vi "Begin.vi"() -> (1 "CameraDevRef":T1)   [LabVIEW 2011]
doc: "Called before other user functions, this VI is expected to open initial I/O refnums, load in file data, and do all program initialization. Notice that the <B>error out</B> terminal is simply used for data flow. Wiring it to other structures or subVIs ensures that this VI runs first."
uses:
  <vilib>/Rock Robotics/WPI/Camera/WPI_CameraDevRef.ctl
  <vilib>/Rock Robotics/SystemInterfaces/DIO/FPGA_DIOPWMChannel.ctl
  <vilib>/Rock Robotics/WPI/Joystick/WPI_JoystickDeviceEnum.ctl
  <vilib>/Rock Robotics/SystemInterfaces/AI/FPGA_AIChannel.ctl
  <vilib>/Rock Robotics/SystemInterfaces/DIO/FPGA_DIORelayChannel.ctl
  <vilib>/Rock Robotics/SystemInterfaces/DIO/FPGA_DIOChannel.ctl
  <vilib>/Rock Robotics/SystemInterfaces/AI/FPGA_AIGyroChannel.ctl
  <vilib>/Rock Robotics/WPI/Encoder/WPI_EncoderType.ctl
  <vilib>/Rock Robotics/WPI/MotorControl/WPI_MotorControlOpen Jaguar.vi
  Robot Global Data.vi
  <vilib>/Utility/file.llb/Read From Spreadsheet File (DBL).vi
  <vilib>/Rock Robotics/WPI/Counter/WPI_CounterDigitalInputToDigitalSource.vi
  <vilib>/Rock Robotics/WPI/RobotDrive/WPI_RobotDriveOpen2MotorWithVictor.vi
  <vilib>/Rock Robotics/WPI/Relay/WPI_RelayDirection.ctl
  <vilib>/Rock Robotics/SystemInterfaces/Typedef/FPGA_TypedefDigitalModule.ctl
  <vilib>/Rock Robotics/SystemInterfaces/Typedef/FPGA_TypedefAnalogModule.ctl
  <vilib>/Rock Robotics/WPI/MotorControl/WPI_MotorControlOpen Victor.vi
panel:
  in  "Minimum Rate":dbl=20.0
  in  "Number Samples to Average":u8=1 min=1 max=128
  in  "DistancePerCount":dbl=1.0
  out "data from file":dbl[](graph)
  in  "Scripted":bool
  out "Path and file":string
  in  "Balls In Robot At Start":dbl
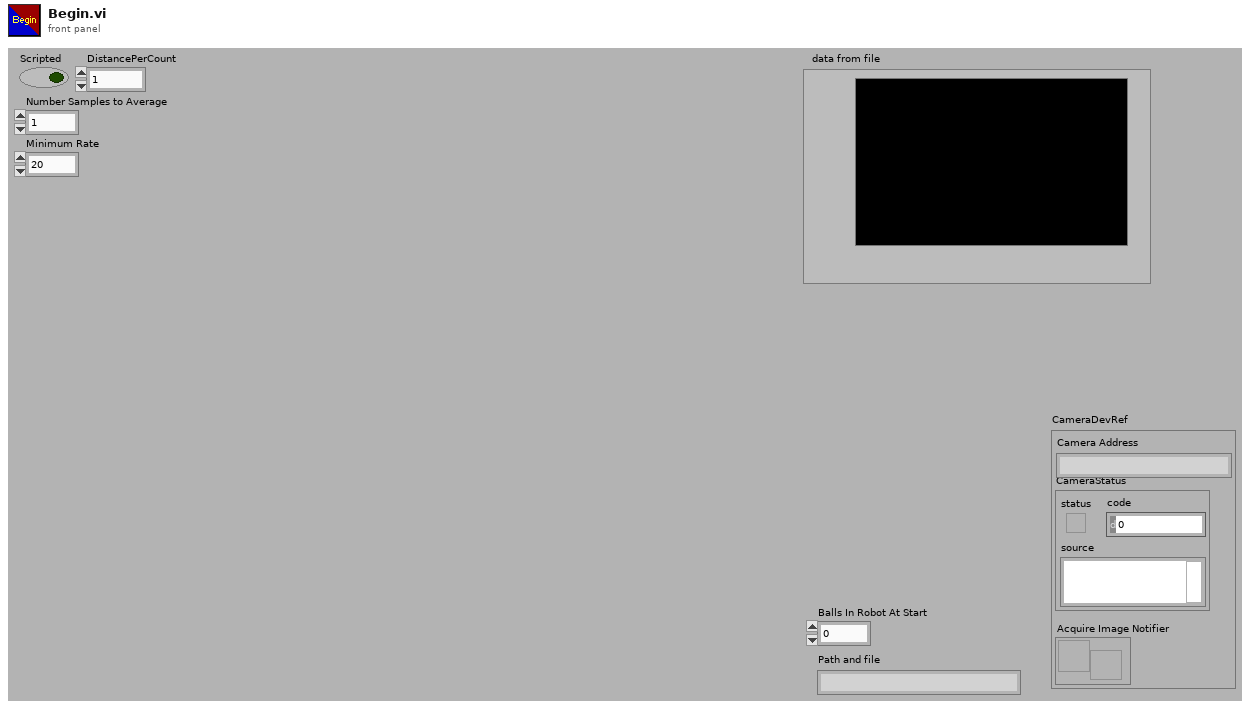
[diagram p1: front panel]
types:
  T1 = typedef "WPI_CameraDevRef.ctl" = cluster{"Camera Address":string, "CameraStatus":errorcluster, "Acquire Image Notifier":refnum<notifier>}
  T2 = typedef "WPI_EncoderType.ctl" = enum16{"1x", "2x", "4x"}
  T3 = typedef "FPGA_DIOChannel.ctl" = enum8{"DIO 1", "DIO 2", "DIO 3", "DIO 4", "DIO 5", "DIO 6", "DIO 7", "DIO 8", "DIO 9", "DIO 10", "DIO 11", "DIO 12", "DIO 13", "DIO 14", "Invalid"}
  T4 = typedef "FPGA_AIGyroChannel.ctl" = enum8{"AI 1", "AI 2", "Invalid"}
  T5 = typedef "FPGA_DIOPWMChannel.ctl" = enum8{"PWM 1", "PWM 2", "PWM 3", "PWM 4", "PWM 5", "PWM 6", "PWM 7", "PWM 8", "PWM 9", "PWM 10", "Invalid"}
  T6 = typedef "FPGA_DIORelayChannel.ctl" = enum8{"Relay 1", "Relay 2", "Relay 3", "Relay 4", "Relay 5", "Relay 6", "Relay 7", "Relay 8", "Invalid"}
  T7 = typedef "FPGA_AIChannel.ctl" = enum8{"AI 1", "AI 2", "AI 3", "AI 4", "AI 5", "AI 6", "AI 7", "AI 8", "Invalid"}
  T8 = typedef "WPI_JoystickDeviceEnum.ctl" = enum16{"USB 1", "USB 2", "USB 3", "USB 4", "Kinect 1", "Kinect 2"}
  T9 = typedef "WPI_MotorControlDeviceRef.ctl" = cluster{"DeviceStatus":errorcluster, "Type":enum16{"PWM", "CAN"}, "PWM":cluster{"Digital Module":T10, "PWM Channel":T5, "DeadBand":T11}, "CAN":cluster{"Device Number":u8, "Control Mode":T12, "Semaphore":T13, "Max Vout":dbl}, "Invert":bool, "TransformRef":T14, "InvTransformRef":T14}
  T10 = typedef "FPGA_TypedefDigitalModule.ctl" = enum16{"Digital Module 1", "Digital Module 2"}
  T11 = typedef "WPI_PWMDeadband.ctl" = cluster{"Name":string, "maxPositivePwm":i32, "minPositivePwm":i32, "centerPwm":i32, "maxNegativePwm":i32, "minNegativePwm":i32, "angularRange":u16}
  T12 = typedef "WPI_CANJaguar_ControlMode.ctl" = enum8{"Percent VBus", "Current", "Speed", "Position", "Voltage"}
  T13 = typedef "Semaphore RefNum" = refnum<k1>
  T14 = typedef "WPI_PWMTransform_ConPane.ctl" = refnum<vi>
  T15 = typedef "WPI_RobotDriveDevRef.ctl" = cluster{"DevStatus":errorcluster, "Motors[]":T9[], "Square Inputs":bool, "Max Output":dbl, "Isochronous":bool}
  T16 = typedef "WPI_CameraImageSize.ctl" = enum16{"640x480", "320x240", "160x120"}
  T17 = cluster{"fps":i32, "compression":i32, "Image Size":T16}
  T18 = typedef "WPI_AnalogChannelDevRef.ctl" = cluster{"DevStatus":errorcluster, "Analog Module":T19, "Analog Channel":T7}
  T19 = typedef "FPGA_TypedefAnalogModule.ctl" = enum16{"Analog Module 1", "Analog Module 2"}
  T20 = typedef "WPI_ServoDeviceRef.ctl" = cluster{"DeviceStatus":errorcluster, "Digital Module":T10, "PWM Channel":T5, "DeadBand":T11}
  T21 = typedef "WPI_CameraWhite Balance Values.ctl" = enum16{"Auto", "Fixed indoor", "Fixed outdoor 1", "Fixed outdoor 2", "Fixed fluorescent 1", "Fixed fluorescent 2", "Hold current"}
  T22 = typedef "WPI_RelayDirection.ctl" = enum16{"Both directions", "Forward only", "Reverse only"}
  T23 = typedef "WPI_RelayDevRef.ctl" = cluster{"DevStatus":errorcluster, "Relay Channel":T6, "Digital Module":T10, "Relay Direction":T22}
  T24 = typedef "WPI_JoystickDevRef.ctl" = cluster{"Device":T8}
  T25 = typedef "WPI_CameraExposure Values.ctl" = enum16{"Auto", "Flicker-free 50 Hz", "Flicker-free 60 Hz", "Hold current"}
  T26 = typedef "WPI_DigitalInputDevRef.ctl" = cluster{"DevStatus":errorcluster, "DIO Channel":T3, "Digital Module":T10}
  T27 = typedef "FPGA_CounterEncoderSourceConvertionLVSourceType.ctl" = cluster{"DevStatus":errorcluster, "AnalogTriggerMode?":bool, "DigitalMode":cluster{"Digital Module":T10, "DIO Channel":T28}, "AnalogTriggerMode":cluster{"AnalogTriggerIndex":T29, "OutputType":T30}}
  T28 = typedef "FPGA_DIODigitalSourceChannel.ctl" = enum8{"DIO 1", "DIO 2", "DIO 3", "DIO 4", "DIO 5", "DIO 6", "DIO 7", "DIO 8", "DIO 9", "DIO 10", "DIO 11", "DIO 12", "DIO 13", "DIO 14", "Disabled"}
  T29 = typedef "FPGA_AnalogTriggerIndex.ctl" = enum8{"Trig 0", "Trig 1", "Trig 2", "Trig 3", "Trig 4", "Trig 5", "Trig 6", "Trig 7", "Invalid"}
  T30 = typedef "FPGA_AnalogTriggerOutType.ctl" = enum16{"InWindow", "TriggerState", "Rising", "Falling"}
  T31 = typedef "WPI_EncoderDevRef.ctl" = cluster{"DevStatus":errorcluster, "EncoderIndex":T32, "CounterIndex":T33, "DistancePerCount":dbl, "Decoding Type":T2}
  T32 = typedef "FPGA_EncoderIdx.ctl" = enum8{"Enc 0", "Enc 1", "Enc 2", "Enc 3", "Invalid"}
  T33 = typedef "FPGA_CounterCtrSystemIndex.ctl" = enum8{"Ctr 0", "Ctr 1", "Ctr 2", "Ctr 3", "Ctr 4", "Ctr 5", "Ctr 6", "Ctr 7", "Invalid"}
  T34 = enum16{"big-endian, network order", "native, host order", "little-endian"}
  T35 = cluster{"[0]":dbl, "[1]":dbl, "[2]":dbl, "[3]":dbl, "[4]":dbl, "[5]":dbl, "[6]":dbl, "[7]":dbl, "[8]":dbl}
  T36 = typedef "WPI_GyroDevRef.ctl" = cluster{"DevStatus":errorcluster, "Analog Module":T19, "Analog Channel":T7, "Offset":dbl, "Gain (VoltsPerDegree/Second)":dbl}
  T37 = typedef "WPI_UltrasonicDeviceRef.ctl" = cluster{"DevStatus":errorcluster, "Ping Digital Module":T10, "Echo Digital Module":T10, "Ping Channel":T3, "Echo Channel":T3, "CntIndex":T33}
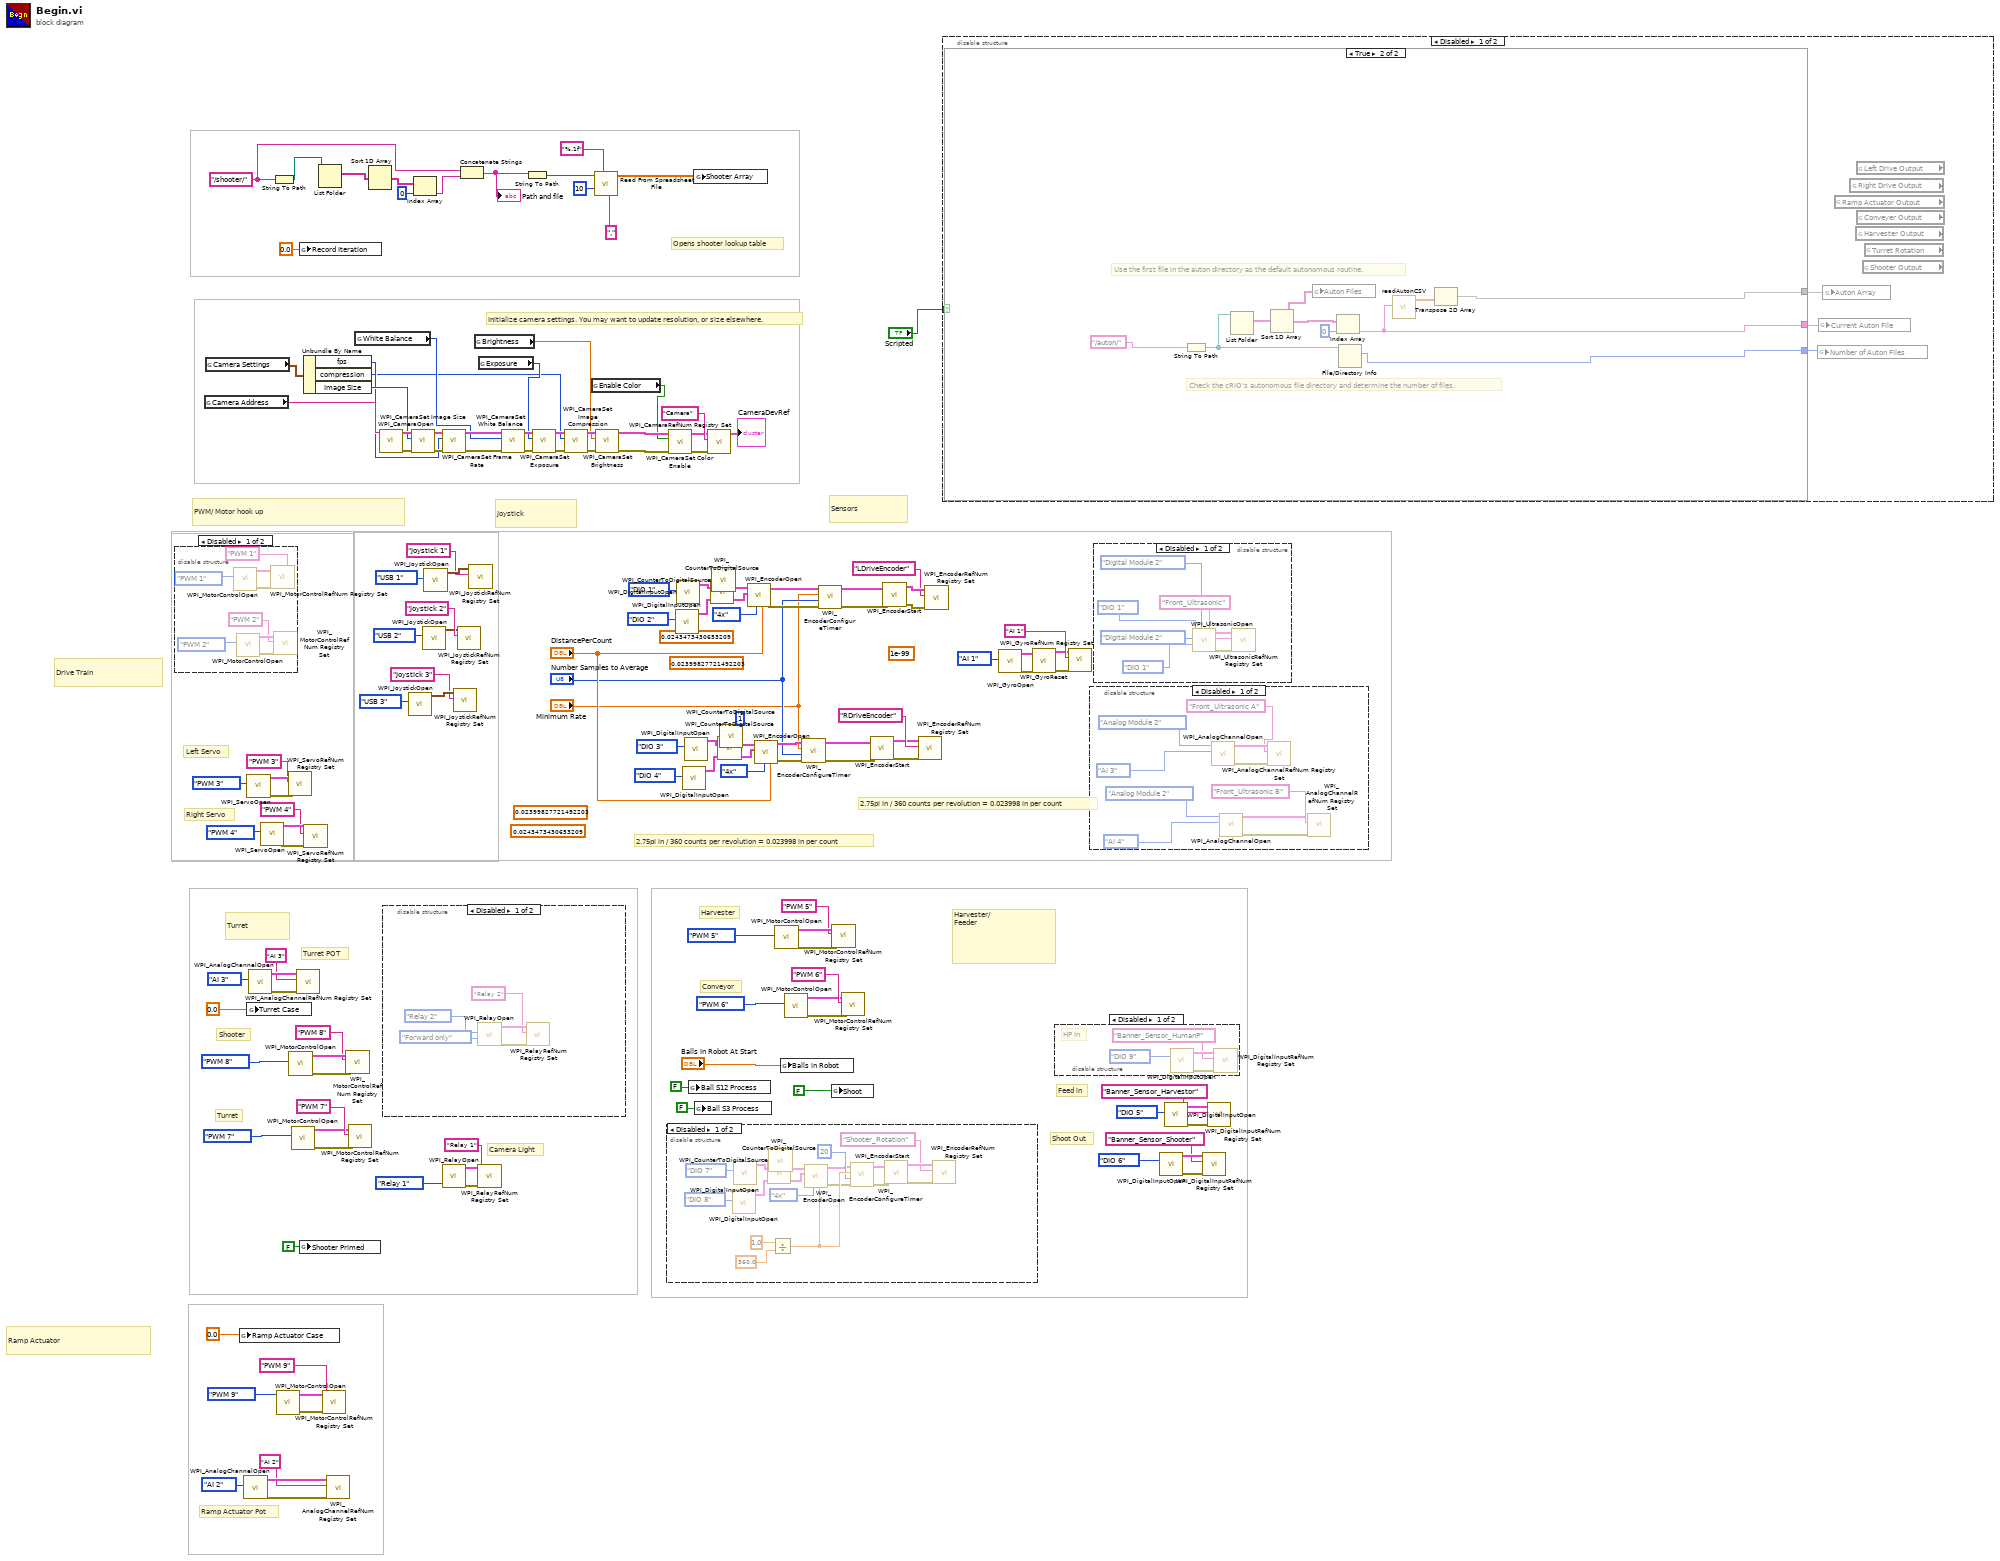
[diagram p0: block diagram]
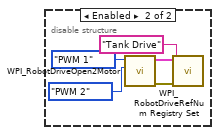
[diagram p2: hidden frame]
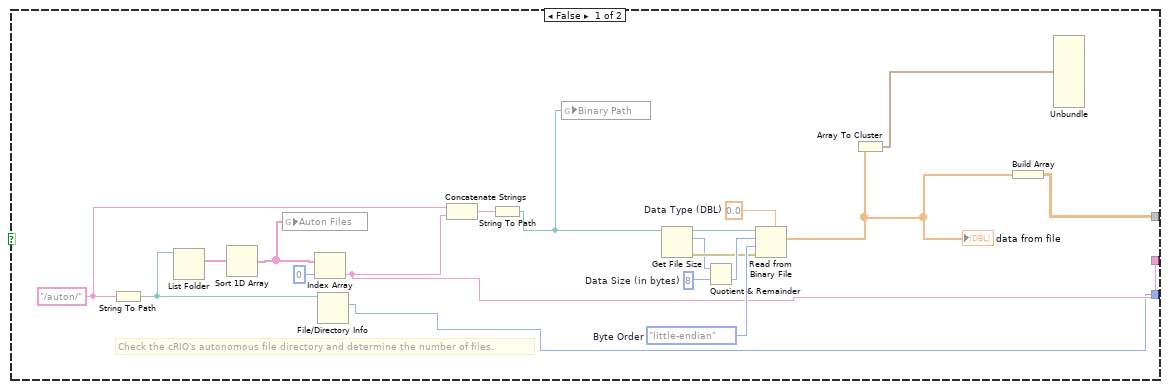
[diagram p3: hidden frame]
diagram:
  (unwired) 1e-99 ("Minimum Rate")
  (unwired) 0.0243473430653209 ("DistancePerCount")
  (unwired) 0.0243473430653209 ("DistancePerCount")
  (unwired) u8 1 ("Number Samples to Average")
  (unwired) 0.02399827721492203 ("DistancePerCount")
  (unwired) 0.02399827721492203 ("DistancePerCount")
  w37 = "/shooter/" ("string")
  # "2.75pi in / 360 counts per revolution = 0.023998 in per count"
  # "2.75pi in / 360 counts per revolution = 0.023998 in per count"
  # "Opens shooter lookup table"
  # "Shoot Out"
  # "Feed in"
  # "Harvester"
  # "Conveyor"
  # "Shooter"
  # "Initialize camera settings. You may want to update resolution, or size elsewhere."
  # "Camera Light"
  # "Ramp Actuator Pot"
  # "Turret POT"
  # "Turret"
  # "Right Servo"
  # "Left Servo"
  # "Harvester/\nFeeder"
  # "Turret"
  # "Ramp Actuator"
  # "Drive Train"
  # "Sensors"
  # "Joystick"
  # "PWM/ Motor hook up"
  n1 = disable-structure shown="Disabled" {
    frame Disabled {
      n2 = call-poly <vilib>:"WPI_MotorControlOpen.vi"("PWM Channel"=FPGA_DIOPWMChannel."PWM 1") -> ("error out"=w148:errorcluster, "MotorControlDeviceRef"=w150:T9)  [unwired: 9 in]
      n3 = call-poly <vilib>:"WPI_MotorControlOpen.vi"("PWM Channel"=FPGA_DIOPWMChannel."PWM 2") -> ("error out"=w146:errorcluster, "MotorControlDeviceRef"=w144:T9)  [unwired: 9 in]
      n4 = call <vilib>:"WPI_MotorControlRefNum Registry Set.vi"("error in (no error)"=w148, "refnum name"="PWM 1", "MotorControlDevRef"=w150) -> ()  [unwired: 7 in, 2 out]
      n5 = call <vilib>:"WPI_MotorControlRefNum Registry Set.vi"("error in (no error)"=w146, "refnum name"="PWM 2", "MotorControlDevRef"=w144) -> ()  [unwired: 7 in, 2 out]
    }
    frame Enabled {
      n6 = call-poly <vilib>:"WPI_RobotDriveOpen2Motor.vi"("Right Motor"=FPGA_DIOPWMChannel."PWM 2", "Left Motor"=FPGA_DIOPWMChannel."PWM 1") -> ("error out"=w155:errorcluster, "RobotDriveDevRef"=w154:T15)  [unwired: 8 in]
      n7 = call <vilib>:"WPI_RobotDriveRefNum Registry Set.vi"("error in (no error)"=w155, "refnum name"="Tank Drive", "RobotDriveDevRef"=w154) -> ()  [unwired: 7 in, 2 out]
    }
  }
  n8 = global read "Robot Global Data.vi" "Camera Address"() -> (w90:string)
  n9 = global read "Robot Global Data.vi" "Camera Settings"() -> (w89:T17)
  n10 = global write "Robot Global Data.vi" "Ramp Actuator Case"(0.0 ("Ramp Actuator Case")) -> ()
  n11 = call <vilib>:"WPI_AnalogChannelOpen.vi"("Analog Channel"=FPGA_AIChannel."AI 2") -> ("error out"=w115:errorcluster, "AIDeviceRef"=w116:T18)  [unwired: 9 in]
  n12 = call <vilib>:"WPI_ServoOpen.vi"("PWM Channel"=FPGA_DIOPWMChannel."PWM 3") -> ("error out"=w136:errorcluster, "ServoDeviceRef"=w141:T20)  [unwired: 9 in]
  n13 = global write "Robot Global Data.vi" "Turret Case"(0.0 ("Return To Home Case")) -> ()
  n14 = call <vilib>:"WPI_AnalogChannelOpen.vi"("Analog Channel"=FPGA_AIChannel."AI 3") -> ("error out"=w120:errorcluster, "AIDeviceRef"=w121:T18)  [unwired: 9 in]
  n15 = call <vilib>:"WPI_ServoOpen.vi"("PWM Channel"=FPGA_DIOPWMChannel."PWM 4") -> ("error out"=w135:errorcluster, "ServoDeviceRef"=w139:T20)  [unwired: 9 in]
  n16 = String To Path(string=w37) -> (path=w46:path)
  n17 = call-poly <vilib>:"WPI_MotorControlOpen.vi"("PWM Channel"=FPGA_DIOPWMChannel."PWM 9") -> ("error out"=w110:errorcluster, "MotorControlDeviceRef"=w111:T9)  [unwired: 9 in]
  n18 = call <vilib>:"WPI_ServoRefNum Registry Set.vi"("error in (no error)"=w136, "refnum name"="PWM 3", "ServoDeviceRef"=w141) -> ()  [unwired: 7 in, 2 out]
  n19 = call-poly <vilib>:"WPI_MotorControlOpen.vi"("PWM Channel"=FPGA_DIOPWMChannel."PWM 8") -> ("error out"=w73:errorcluster, "MotorControlDeviceRef"=w75:T9)  [unwired: 9 in]
  n20 = call-poly <vilib>:"WPI_MotorControlOpen.vi"("PWM Channel"=FPGA_DIOPWMChannel."PWM 7") -> ("error out"=w125:errorcluster, "MotorControlDeviceRef"=w123:T9)  [unwired: 9 in]
  n21 = call <vilib>:"WPI_AnalogChannelRefNum Registry Set.vi"("error in (no error)"=w120, "refnum name"="AI 3", "AIDeviceRef"=w121) -> ()  [unwired: 7 in, 2 out]
  n22 = global write "Robot Global Data.vi" "Record Iteration"(0.0 ("Record Iteration")) -> ()
  n23 = global write "Robot Global Data.vi" "Shooter Primed"(FALSE ("Ball S3 Process")) -> ()
  n24 = Unbundle By Name(w89) -> ("fps"=w87:i32, "compression"=w84:i32, "Image Size"=w88:T16)
  n25 = call <vilib>:"WPI_ServoRefNum Registry Set.vi"("error in (no error)"=w135, "refnum name"="PWM 4", "ServoDeviceRef"=w139) -> ()  [unwired: 7 in, 2 out]
  n26 = List Folder(path=w46) -> (filenames=w45:string[])  [unwired: 1 in, 5 out]
  n27 = call <vilib>:"WPI_MotorControlRefNum Registry Set.vi"("error in (no error)"=w110, "refnum name"="PWM 9", "MotorControlDevRef"=w111) -> ()  [unwired: 7 in, 2 out]
  n28 = call <vilib>:"WPI_AnalogChannelRefNum Registry Set.vi"("error in (no error)"=w115, "refnum name"="AI 2", "AIDeviceRef"=w116) -> ()  [unwired: 7 in, 2 out]
  n29 = call <vilib>:"WPI_MotorControlRefNum Registry Set.vi"("error in (no error)"=w73, "refnum name"="PWM 8", "MotorControlDevRef"=w75) -> ()  [unwired: 7 in, 2 out]
  n30 = call <vilib>:"WPI_MotorControlRefNum Registry Set.vi"("error in (no error)"=w125, "refnum name"="PWM 7", "MotorControlDevRef"=w123) -> ()  [unwired: 7 in, 2 out]
  n31 = global read "Robot Global Data.vi" "White Balance"() -> (w86:T21)
  n32 = Sort 1D Array(array=w45) -> (sorted array=w44:string[])
  n33 = call <vilib>:"WPI_CameraOpen.vi"("Camera Address"=w90) -> ("error out"=w96:errorcluster, "CameraDevRef"=w97:T1)  [unwired: 1 in, 8 out]
  n34 = disable-structure shown="Disabled" {
    frame Disabled {
      n35 = call <vilib>:"WPI_RelayOpen.vi"("Relay Direction"=WPI_RelayDirection."Forward only", "Relay Channel"=FPGA_DIORelayChannel."Relay 2") -> ("error out"=w159:errorcluster, "RelayDevRef"=w160:T23)  [unwired: 8 in]
      n36 = call <vilib>:"WPI_RelayRefNum Registry Set.vi"("error in (no error)"=w159, "refnum name"="Relay 2", "RelayDevRef"=w160) -> ()  [unwired: 7 in, 2 out]
    }
    frame Enabled {
    }
  }
  n37 = call <vilib>:"WPI_JoystickOpen.vi"("JoystickDevice"=WPI_JoystickDeviceEnum."USB 3") -> ("JoystickDevRef"=w128:T24)  [unwired: 10 in]
  n38 = call <vilib>:"WPI_CameraSet Image Size.vi"("error in (no error)"=w96, "Image Size"=w88, "CameraDevRef"=w97) -> ("error out"=w95:errorcluster, "CameraDevRef Out"=w98:T1)  [unwired: 7 out]
  n39 = Index Array(array=w44, index=0) -> (element=w36:string)
  n40 = call <vilib>:"WPI_JoystickOpen.vi"("JoystickDevice"=WPI_JoystickDeviceEnum."USB 2") -> ("JoystickDevRef"=w131:T24)  [unwired: 10 in]
  n41 = call <vilib>:"WPI_JoystickOpen.vi"("JoystickDevice"=WPI_JoystickDeviceEnum."USB 1") -> ("JoystickDevRef"=w134:T24)  [unwired: 10 in]
  n42 = call <vilib>:"WPI_CameraSet Frame Rate.vi"("error in (no error)"=w95, "Frame Rate (fps)"=w87, "CameraDevRef"=w98) -> ("error out"=w94:errorcluster, "CameraDevRef Out"=w100:T1)  [unwired: 7 out]
  n43 = call <vilib>:"WPI_RelayOpen.vi"("Relay Channel"=FPGA_DIORelayChannel."Relay 1") -> ("error out"=w107:errorcluster, "RelayDevRef"=w106:T23)  [unwired: 9 in]
  n44 = call <vilib>:"WPI_JoystickRefNum Registry Set.vi"("refnum name"="Joystick 3", "JoystickDevRef"=w128) -> ()  [unwired: 8 in, 2 out]
  n45 = call <vilib>:"WPI_JoystickRefNum Registry Set.vi"("refnum name"="Joystick 2", "JoystickDevRef"=w131) -> ()  [unwired: 8 in, 2 out]
  n46 = Concatenate Strings(w37, w36) -> (w39:string)
  "Path and file" <- w39
  n47 = call <vilib>:"WPI_JoystickRefNum Registry Set.vi"("refnum name"="Joystick 1", "JoystickDevRef"=w134) -> ()  [unwired: 8 in, 2 out]
  n48 = global read "Robot Global Data.vi" "Brightness"() -> (w83:dbl)
  n49 = call <vilib>:"WPI_RelayRefNum Registry Set.vi"("error in (no error)"=w107, "refnum name"="Relay 1", "RelayDevRef"=w106) -> ()  [unwired: 7 in, 2 out]
  n50 = global read "Robot Global Data.vi" "Exposure"() -> (w85:T25)
  n51 = call <vilib>:"WPI_CameraSet White Balance.vi"("error in (no error)"=w94, "White Balance"=w86, "CameraDevRef"=w100) -> ("error out"=w93:errorcluster, "CameraDevRef Out"=w99:T1)  [unwired: 7 out]
  n52 = String To Path(string=w39) -> (path=w38:path)
  n53 = call <vilib>:"WPI_CameraSet Exposure.vi"("error in (no error)"=w93, "Exposure"=w85, "CameraDevRef"=w99) -> ("error out"=w92:errorcluster, "CameraDevRef Out"=w102:T1)  [unwired: 7 out]
  n54 = call <vilib>:"WPI_CameraSet Image Compression.vi"("error in (no error)"=w92, "Compression"=w84, "CameraDevRef"=w102) -> ("error out"=w91:errorcluster, "CameraDevRef Out"=w101:T1)  [unwired: 7 out]
  n55 = global read "Robot Global Data.vi" "Enable Color"() -> (w78:bool)
  n56 = call-poly <vilib>:"Read From Spreadsheet File.vi"("delimiter (\\t)"="," ("delimiter (\\t)"), "format (%.3f)"="%.1f", "number of rows (all:-1)"=10, "file path (dialog if empty)"=w38) -> ("all rows"=w35:dbl[][])  [unwired: 1 in, 6 out]
  n57 = call <vilib>:"WPI_CameraSet Brightness.vi"("error in (no error)"=w91, "Brightness"=w83, "CameraDevRef"=w101) -> ("error out"=w81:errorcluster, "CameraDevRef Out"=w82:T1)  [unwired: 7 out]
  n58 = disable-structure shown="Disabled" {
    frame Disabled {
      n59 = call <vilib>:"WPI_DigitalInputOpen.vi"("DIO Channel"=FPGA_DIOChannel."DIO 8") -> ("DigitalInputDevRef"=w165:T26)  [unwired: 9 in, 1 out]
      n60 = call <vilib>:"WPI_DigitalInputOpen.vi"("DIO Channel"=FPGA_DIOChannel."DIO 7") -> ("DigitalInputDevRef"=w162:T26)  [unwired: 9 in, 1 out]
      n61 = call-poly <vilib>:"WPI_CounterToDigitalSource.vi"("DigitalInputDevRef"=w165) -> ("Digital Source"=w166:T27)  [unwired: 6 in]
      n62 = call-poly <vilib>:"WPI_CounterToDigitalSource.vi"("DigitalInputDevRef"=w162) -> ("Digital Source"=w161:T27)  [unwired: 6 in]
      n63 = Divide(x=1.0, y=360.0) -> (x/y=w178:dbl)
      n64 = call <vilib>:"WPI_EncoderOpen.vi"("DistancePerCount"=w178, "Decoding Type"=WPI_EncoderType."4x", "BSource"=w166, "ASource"=w161) -> ("error out"=w169:errorcluster, "EncoderDevRef"=w170:T31)  [unwired: 6 in]
      n65 = call <vilib>:"WPI_EncoderConfigureTimer.vi"("error in (no error)"=w169, "Number Samples to Average"=u8 20, "Minimum Rate"=w178, "EncoderDevRef"=w170) -> ("error out"=w173:errorcluster, "EncoderDevRef"=w172:T31)  [unwired: 6 in]
      n66 = call <vilib>:"WPI_EncoderStart.vi"("error in (no error)"=w173, "EncoderDevRef"=w172) -> ("error out"=w175:errorcluster, "EncoderDevRef"=w174:T31)  [unwired: 8 in]
      n67 = call <vilib>:"WPI_EncoderRefNum Registry Set.vi"("error in (no error)"=w175, "refnum name"="Shooter_Rotation", "EncoderDevRef"=w174) -> ()  [unwired: 7 in, 2 out]
    }
    frame Enabled {
    }
  }
  n68 = call <vilib>:"WPI_CameraSet Color Enable.vi"("error in (no error)"=w81, "Color Enabled"=w78, "CameraDevRef"=w82) -> ("error out"=w79:errorcluster, "CameraDevRef Out"=w80:T1)  [unwired: 7 in]
  n69 = call <vilib>:"WPI_DigitalInputOpen.vi"("DIO Channel"=FPGA_DIOChannel."DIO 2") -> ("DigitalInputDevRef"=w27:T26)  [unwired: 9 in, 1 out]
  n70 = call <vilib>:"WPI_DigitalInputOpen.vi"("DIO Channel"=FPGA_DIOChannel."DIO 1") -> ("DigitalInputDevRef"=w24:T26)  [unwired: 9 in, 1 out]
  n71 = call <vilib>:"WPI_DigitalInputOpen.vi"("DIO Channel"=FPGA_DIOChannel."DIO 4") -> ("DigitalInputDevRef"=w18:T26)  [unwired: 9 in, 1 out]
  n72 = call <vilib>:"WPI_DigitalInputOpen.vi"("DIO Channel"=FPGA_DIOChannel."DIO 3") -> ("DigitalInputDevRef"=w21:T26)  [unwired: 9 in, 1 out]
  n73 = global write "Robot Global Data.vi" "Ball S12 Process"(FALSE ("Ball S12 Process")) -> ()
  n74 = global write "Robot Global Data.vi" "Shooter Array"(w35) -> ()
  n75 = global write "Robot Global Data.vi" "Ball S3 Process"(FALSE ("Ball S3 Process")) -> ()
  n76 = call <vilib>:"WPI_CameraRefNum Registry Set.vi"("error in (no error)"=w79, "refnum name"="Camera", "CameraDevRef"=w80) -> ("CameraDevRef"=→"CameraDevRef":T1)  [unwired: 8 out]
  n77 = call-poly <vilib>:"WPI_CounterToDigitalSource.vi"("DigitalInputDevRef"=w27) -> ("Digital Source"=w28:T27)  [unwired: 6 in]
  n78 = call-poly <vilib>:"WPI_CounterToDigitalSource.vi"("DigitalInputDevRef"=w24) -> ("Digital Source"=w23:T27)  [unwired: 6 in]
  n79 = call-poly <vilib>:"WPI_CounterToDigitalSource.vi"("DigitalInputDevRef"=w18) -> ("Digital Source"=w17:T27)  [unwired: 6 in]
  n80 = call-poly <vilib>:"WPI_CounterToDigitalSource.vi"("DigitalInputDevRef"=w21) -> ("Digital Source"=w22:T27)  [unwired: 6 in]
  n81 = call <vilib>:"WPI_EncoderOpen.vi"("DistancePerCount"="DistancePerCount", "Decoding Type"=WPI_EncoderType."4x", "BSource"=w28, "ASource"=w23) -> ("error out"=w6:errorcluster, "EncoderDevRef"=w7:T31)  [unwired: 6 in]
  n82 = call <vilib>:"WPI_EncoderOpen.vi"("DistancePerCount"="DistancePerCount", "Decoding Type"=WPI_EncoderType."4x", "BSource"=w17, "ASource"=w22) -> ("error out"=w14:errorcluster, "EncoderDevRef"=w13:T31)  [unwired: 6 in]
  n83 = call-poly <vilib>:"WPI_MotorControlOpen.vi"("PWM Channel"=FPGA_DIOPWMChannel."PWM 5") -> ("error out"=w69:errorcluster, "MotorControlDeviceRef"=w71:T9)  [unwired: 9 in]
  n84 = global write "Robot Global Data.vi" "Balls in Robot"("Balls In Robot At Start") -> ()
  n85 = call-poly <vilib>:"WPI_MotorControlOpen.vi"("PWM Channel"=FPGA_DIOPWMChannel."PWM 6") -> ("error out"=w68:errorcluster, "MotorControlDeviceRef"=w66:T9)  [unwired: 9 in]
  n86 = call <vilib>:"WPI_EncoderConfigureTimer.vi"("error in (no error)"=w14, "Number Samples to Average"="Number Samples to Average", "Minimum Rate"="Minimum Rate", "EncoderDevRef"=w13) -> ("error out"=w11:errorcluster, "EncoderDevRef"=w12:T31)  [unwired: 6 in]
  n87 = call <vilib>:"WPI_EncoderConfigureTimer.vi"("error in (no error)"=w6, "Number Samples to Average"="Number Samples to Average", "Minimum Rate"="Minimum Rate", "EncoderDevRef"=w7) -> ("error out"=w5:errorcluster, "EncoderDevRef"=w4:T31)  [unwired: 6 in]
  n88 = global write "Robot Global Data.vi" "Shoot"(FALSE ("Ball S12 Process")) -> ()
  n89 = call <vilib>:"WPI_MotorControlRefNum Registry Set.vi"("error in (no error)"=w69, "refnum name"="PWM 5", "MotorControlDevRef"=w71) -> ()  [unwired: 7 in, 2 out]
  n90 = call <vilib>:"WPI_MotorControlRefNum Registry Set.vi"("error in (no error)"=w68, "refnum name"="PWM 6", "MotorControlDevRef"=w66) -> ()  [unwired: 7 in, 2 out]
  n91 = call <vilib>:"WPI_EncoderStart.vi"("error in (no error)"=w11, "EncoderDevRef"=w12) -> ("error out"=w9:errorcluster, "EncoderDevRef"=w10:T31)  [unwired: 8 in]
  n92 = call <vilib>:"WPI_EncoderStart.vi"("error in (no error)"=w5, "EncoderDevRef"=w4) -> ("error out"=w31:errorcluster, "EncoderDevRef"=w30:T31)  [unwired: 8 in]
  n93 = call <vilib>:"WPI_EncoderRefNum Registry Set.vi"("error in (no error)"=w9, "refnum name"="RDriveEncoder", "EncoderDevRef"=w10) -> ()  [unwired: 7 in, 2 out]
  n94 = call <vilib>:"WPI_EncoderRefNum Registry Set.vi"("error in (no error)"=w31, "refnum name"="LDriveEncoder", "EncoderDevRef"=w30) -> ()  [unwired: 7 in, 2 out]
  n95 = disable-structure shown="Disabled" {
    disable-tunnel: "Scripted" -> [w182 _]
    frame Disabled {
      n96 = case shown="True" w182 {
        tunnel: [w185 w210] -> w181
        tunnel: [w186 w209] -> w180
        tunnel: [w187 w208] -> w179
        frame False {
          w195 = T34."little-endian"  # Byte Order
          w193 = i64 8  # Data Size (in bytes)
          w192 = 0.0  # Data Type (DBL)
          w200 = "/auton/" ("string")
          # "Check the cRIO's autonomous file directory and determine the number of files."
          n97 = String To Path(string=w200) -> (path=w196:path)
          n98 = List Folder(path=w196) -> (filenames=w197:string[])  [unwired: 1 in, 5 out]
          n99 = Sort 1D Array(array=w197) -> (sorted array=w199:string[])
          n100 = global write "Robot Global Data.vi" "Auton Files"(w199) -> ()
          n101 = Index Array(array=w199, index=0) -> (element=w186:string)
          n102 = File/Directory Info(path=w196) -> (size=w185:i64)  [unwired: 1 in, 6 out]
          n103 = Concatenate Strings(w200, w186) -> (w201:string)
          n104 = String To Path(string=w201) -> (path=w188:path)
          n105 = global write "Robot Global Data.vi" "Binary Path"(w188) -> ()
          n106 = Get File Size(file=w188) -> (refnum out=w189:refnum<file>, size (in bytes)=w190:i64, 0:w191:errorcluster)  [unwired: 1 in]
          n107 = Quotient & Remainder(x=w190, y=w193) -> (floor(x/y)=w194:i64)  [unwired: 1 out]
          n108 = Read from Binary File(5:w192, 8:w191, 9:w195, 10:w194, 11:w189) -> (2:w183:dbl[])  [unwired: 1 in, 3 out]
          "data from file" <- w183
          n109 = Array To Cluster(array=w183) -> (cluster=w184:T35)
          n110 = Build Array(w183) -> (w187:dbl[][])
          n111 = Unbundle(w184) -> ()  [unwired: 9 out]
        }
        frame True {
          # "Check the cRIO's autonomous file directory and determine the number of files."
          # "Use the first file in the auton directory as the default autonomous routine."
          n112 = String To Path(string="/auton/") -> (path=w206:path)
          n113 = List Folder(path=w206) -> (filenames=w205:string[])  [unwired: 1 in, 5 out]
          n114 = Sort 1D Array(array=w205) -> (sorted array=w203:string[])
          n115 = global write "Robot Global Data.vi" "Auton Files"(w203) -> ()
          n116 = Index Array(array=w203, index=0) -> (element=w209:string)
          n117 = File/Directory Info(path=w206) -> (size=w210:i64)  [unwired: 1 in, 6 out]
          n118 = call "readAutonCSV.vi"("AutonFile"=w209) -> ("AutonArray"=w202:dbl[][])  [unwired: 7 in]
          n119 = Transpose 2D Array(2D array=w202) -> (transposed array=w208:dbl[][])
        }
      }
      n120 = global write "Robot Global Data.vi" "Number of Auton Files"(w181) -> ()
      n121 = global write "Robot Global Data.vi" "Current Auton File"(w180) -> ()
      n122 = global write "Robot Global Data.vi" "Auton Array"(w179) -> ()
      n123 = global read "Robot Global Data.vi" "Ramp Actuator Output"() -> ()  [unwired: 1 out]
      n124 = global read "Robot Global Data.vi" "Right Drive Output"() -> ()  [unwired: 1 out]
      n125 = global read "Robot Global Data.vi" "Harvester Output"() -> ()  [unwired: 1 out]
      n126 = global read "Robot Global Data.vi" "Left Drive Output"() -> ()  [unwired: 1 out]
      n127 = global read "Robot Global Data.vi" "Conveyer Output"() -> ()  [unwired: 1 out]
      n128 = global read "Robot Global Data.vi" "Shooter Output"() -> ()  [unwired: 1 out]
      n129 = global read "Robot Global Data.vi" "Turret Rotation"() -> ()  [unwired: 1 out]
    }
    frame Enabled {
    }
  }
  n130 = call <vilib>:"WPI_GyroOpen.vi"("Analog Channel"=FPGA_AIGyroChannel."AI 1") -> ("error out"=w49:errorcluster, "GyroDevRef"=w50:T36)  [unwired: 8 in, 1 out]
  n131 = call <vilib>:"WPI_GyroReset.vi"("error in (no error)"=w49, "GyroDevRef"=w50) -> ("error out"=w48:errorcluster, "GyroDevRef"=w47:T36)  [unwired: 8 in]
  n132 = disable-structure shown="Disabled" {
    frame Disabled {
      # "HP In"
      n133 = call <vilib>:"WPI_DigitalInputOpen.vi"("DIO Channel"=FPGA_DIOChannel."DIO 9") -> ("error out"=w213:errorcluster, "DigitalInputDevRef"=w212:T26)  [unwired: 9 in]
      n134 = call <vilib>:"WPI_DigitalInputRefNum Registry Set.vi"("error in (no error)"=w213, "refnum name"="Banner_Sensor_HumanP", "DigitalInputDevRef"=w212) -> ()  [unwired: 7 in, 2 out]
    }
    frame Enabled {
    }
  }
  n135 = call <vilib>:"WPI_GyroRefNum Registry Set.vi"("error in (no error)"=w48, "refnum name"="AI 1", "GyroDevRef"=w47) -> ()  [unwired: 7 in, 2 out]
  n136 = disable-structure shown="Disabled" {
    frame Disabled {
      n137 = call <vilib>:"WPI_AnalogChannelOpen.vi"("Analog Channel"=FPGA_AIChannel."AI 3", "Analog Module (Module 1)"=FPGA_TypedefAnalogModule."Analog Module 2") -> ("error out"=w220:errorcluster, "AIDeviceRef"=w219:T18)  [unwired: 8 in]
      n138 = call <vilib>:"WPI_AnalogChannelOpen.vi"("Analog Channel"=FPGA_AIChannel."AI 4", "Analog Module (Module 1)"=FPGA_TypedefAnalogModule."Analog Module 2") -> ("error out"=w215:errorcluster, "AIDeviceRef"=w216:T18)  [unwired: 8 in]
      n139 = call <vilib>:"WPI_AnalogChannelRefNum Registry Set.vi"("error in (no error)"=w220, "refnum name"="Front_Ultrasonic A", "AIDeviceRef"=w219) -> ()  [unwired: 7 in, 2 out]
      n140 = call <vilib>:"WPI_AnalogChannelRefNum Registry Set.vi"("error in (no error)"=w215, "refnum name"="Front_Ultrasonic B", "AIDeviceRef"=w216) -> ()  [unwired: 7 in, 2 out]
    }
    frame Enabled {
    }
  }
  n141 = disable-structure shown="Disabled" {
    frame Disabled {
      n142 = call <vilib>:"WPI_UltrasonicOpen.vi"("Ping Digital Module (Module 1)"=FPGA_TypedefDigitalModule."Digital Module 2", "Echo DIO Channel"=FPGA_DIOChannel."DIO 1", "Echo Digital Module (Module 1)"=FPGA_TypedefDigitalModule."Digital Module 2", "Ping DIO Channel"=FPGA_DIOChannel."DIO 1") -> ("error out"=w231:errorcluster, "UltrasonicDevRef"=w230:T37)  [unwired: 6 in]
      n143 = call <vilib>:"WPI_UltrasonicRefNum Registry Set.vi"("error in (no error)"=w231, "refnum name"="Front_Ultrasonic", "UltrasonicDevRef"=w230) -> ()  [unwired: 7 in, 2 out]
    }
    frame Enabled {
    }
  }
  n144 = call <vilib>:"WPI_DigitalInputOpen.vi"("DIO Channel"=FPGA_DIOChannel."DIO 6") -> ("error out"=w59:errorcluster, "DigitalInputDevRef"=w58:T26)  [unwired: 9 in]
  n145 = call <vilib>:"WPI_DigitalInputOpen.vi"("DIO Channel"=FPGA_DIOChannel."DIO 5") -> ("error out"=w62:errorcluster, "DigitalInputDevRef"=w61:T26)  [unwired: 9 in]
  n146 = call <vilib>:"WPI_DigitalInputRefNum Registry Set.vi"("error in (no error)"=w59, "refnum name"="Banner_Sensor_Shooter", "DigitalInputDevRef"=w58) -> ()  [unwired: 7 in, 2 out]
  n147 = call <vilib>:"WPI_DigitalInputRefNum Registry Set.vi"("error in (no error)"=w62, "refnum name"="Banner_Sensor_Harvestor", "DigitalInputDevRef"=w61) -> ()  [unwired: 7 in, 2 out]
